vi "Laser Power Ctrl Set Caption.vi"(2 "Caption Text":string, 7 "Setup Controls":refnum<vi>[](array[refnum])) -> ()   [LabVIEW 2016]
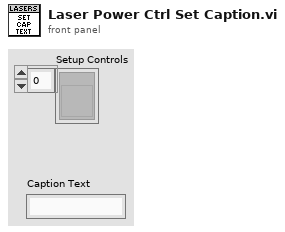
[diagram p1: front panel]
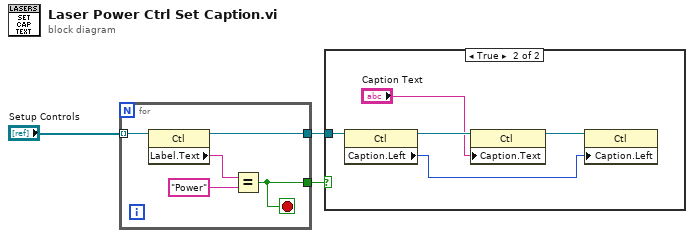
[diagram p0: block diagram]
diagram:
  n1 = for {
    tunnel: "Setup Controls" -> [w8] mode=indexing
    tunnel: [w5] -> w3
    tunnel: [w4] -> w2
    stop <- w5 stop-if-true
    n2 = property class="Ctl"(reference=w8) -> (reference out=w4:refnum<vi>, "Label.Text"=w7:string)  [unwired: 1 in, 1 out]
    n3 = Equal?(x=w7, y="Power") -> (x = y?=w5:bool)
  }
  n4 = case shown="True" w3 {
    tunnel: w2 -> [_ w13]
    frame False {
    }
    frame True {
      n5 = property class="Ctl"(reference=w13) -> (reference out=w12:refnum<vi>, "Caption.Left"=w10:i32)  [unwired: 1 in, 1 out]
      n6 = property class="Ctl"(reference=w12, "Caption.Text"="Caption Text") -> (reference out=w11:refnum<vi>)  [unwired: 1 in, 1 out]
      n7 = property class="Ctl"(reference=w11, "Caption.Left"=w10) -> ()  [unwired: 1 in, 2 out]
    }
  }
